vi "motorPwm.vi"(7 "reverse?":bool, 8 "error in (no error)":errorcluster, 10 "Speed (PWM)":dbl) -> (0 "error out":errorcluster)   [LabVIEW 2019, in "SJCube_ElvisIII.lvlib"]
uses:
  SJCube_ElvisIII.lvlib
  <vilib>/myRIO/Express VI/Onboard IO/PWM/PWM Express VI.xnode
  <vilib>/myRIO/Common/Instrument Driver Framework/Utilities/typedefs/myRIO Generic Hardware Reference.ctl
  <vilib>/myRIO/Common/Instrument Driver Framework/Utilities/typedefs/myRIO v1.0 Reference.ctl
  <vilib>/myRIO/Common/Instrument Driver Framework/Utilities/typedefs/Generic FPGA Reference.ctl
  <vilib>/myRIO/Common/Instrument Driver Framework/Utilities/typedefs/Hardware Version Enum.ctl
  <vilib>/userDefined/High Color/nirio_resource_hc.ctl
  <vilib>/myRIO/Common/Instrument Driver Framework/Utilities/vis/Is FPGA Ref Available.vi
  <vilib>/myRIO/Express VI/Onboard IO/DO/DO Express VI.xnode
  <vilib>/myRIO/Instrument Drivers/Onboard IO/DIO/typedefs/DIO Reference.ctl
  <vilib>/myRIO/Instrument Drivers/Onboard IO/DIO/DIO.lvlib
  <vilib>/myRIO/Common/Instrument Driver Framework/myRIO v1.0/DIO/typedefs/DIO Channels List.ctl
  <vilib>/myRIO/Common/Instrument Driver Framework/myRIO v1.0/DIO/typedefs/DIO Channels Enum.ctl
  <vilib>/myRIO/Instrument Drivers/Onboard IO/DIO/vis/Write.vi
  <vilib>/myRIO/Instrument Drivers/Onboard IO/DIO/vis/myRIO DIO Open.xnode
  <vilib>/myRIO/Common/Instrument Driver Framework/ELVIS III v1.0/DIO/vis/ELVIS III v1.1 Open DIO.vi
  <vilib>/myRIO/Instrument Drivers/Onboard IO/PWM/vis/Set Duty Cycle and Frequency.vi
  <vilib>/myRIO/Instrument Drivers/Onboard IO/PWM/PWM.lvlib
  <vilib>/myRIO/Instrument Drivers/Onboard IO/PWM/typedefs/PWM Configuration.ctl
  <vilib>/myRIO/Common/Instrument Driver Framework/myRIO v1.0/PWM/typedefs/PWM Channels Enum.ctl
  <vilib>/myRIO/Instrument Drivers/Onboard IO/PWM/typedefs/PWM Reference.ctl
  <vilib>/myRIO/Instrument Drivers/Onboard IO/PWM/vis/myRIO PWM Open.xnode
  <vilib>/myRIO/Common/Instrument Driver Framework/ELVIS III v1.0/PWM/vis/ELVIS III v1.1 Open PWM.vi
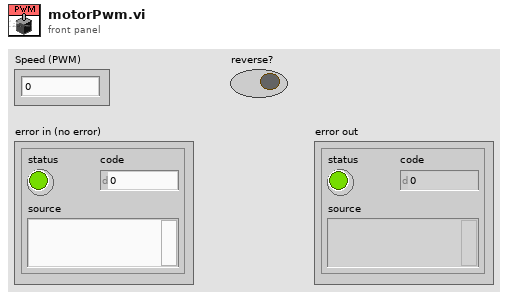
[diagram p1: front panel]
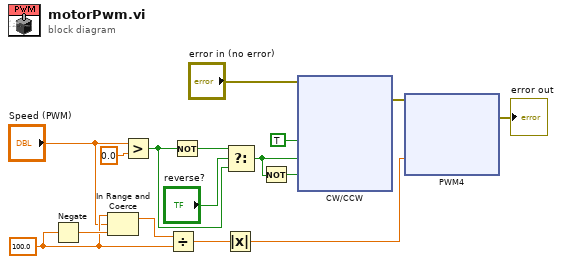
[diagram p0: block diagram]
diagram:
  w14 = 100.0 ("upper limit")
  n1 = Negate(x=w14) -> (-x=w15:dbl)
  n2 = In Range and Coerce(upper limit=w14, x="Speed (PWM)", lower limit=w15) -> (coerced(x)=w16:dbl)  [unwired: 1 out]
  n3 = Greater?(x="Speed (PWM)", y=0.0) -> (0:w2:bool)
  n4 = Divide(x=w16, y=w14) -> (x/y=w13:dbl)
  n5 = Not(x=w2) -> (.not. x?=w3:bool)
  n6 = Absolute Value(x=w13) -> (abs(x)=w12:dbl)
  n7 = Select(t=w3, s="reverse?", f=w2) -> (s? t:f=w1:bool)
  n8 = Not(x=w1) -> (.not. x?=w6:bool)
  n9 = xnode "CW/CCW"("EN (A/DIO5)"=TRUE, "INA (A/DIO6)"=w1, "INB (A/DIO7)"=w6, "error in (no error)"="error in (no error)") -> ("error out"=w8:errorcluster)
  n10 = xnode "PWM4"("Duty Cycle"=w12, "error in (no error)"=w8) -> ("error out"=→"error out":errorcluster)
